vi "ConvDsbAM+_SubVI_.vi"(6 "Modulation Index":dbl, 9 "Carrier Freq":dbl, 10 "sampling info":cluster{"Fs":dbl, "#s":dbl}, 11 "Modullation Freq":dbl) -> (3 "Waveform":waveform(dbl))   [LabVIEW 2011]
uses:
  <vilib>/measure/NI_MABase.lvlib
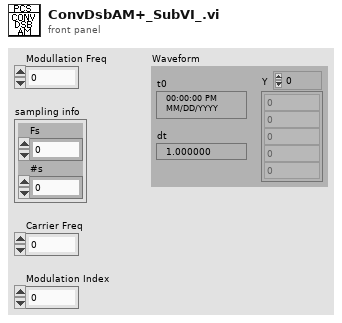
[diagram p1: front panel]
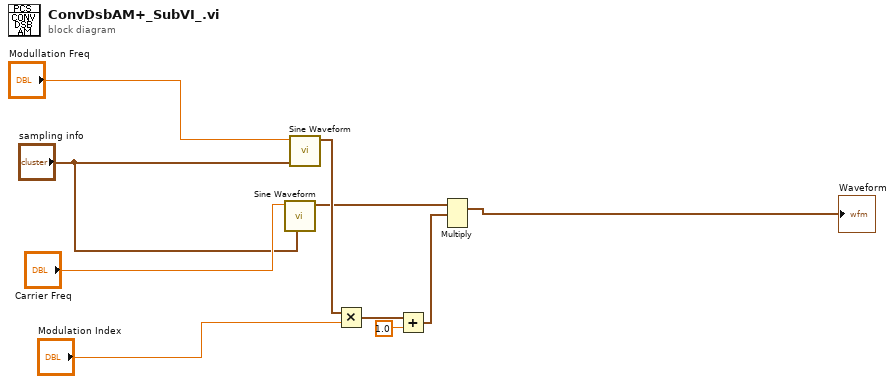
[diagram p0: block diagram]
diagram:
  n1 = call <vilib>:"Sine Waveform.vi"("sampling info"="sampling info", "frequency"="Carrier Freq") -> ("signal out"=w5:waveform(dbl))  [unwired: 8 in, 1 out]
  n2 = call <vilib>:"Sine Waveform.vi"("sampling info"="sampling info", "frequency"="Modullation Freq") -> ("signal out"=w9:waveform(dbl))  [unwired: 8 in, 1 out]
  n3 = Multiply(x=w9, y="Modulation Index") -> (x*y=w8:waveform(dbl))
  n4 = Add(x=w8, y=1.0) -> (x+y=w6:waveform(dbl))
  n5 = Multiply(1:w6, 2:w5) -> (0:→"Waveform":waveform(dbl))  [unwired: 1 in, 1 out]
